vi "HandleObservationSync.vi"(8 "error in (no error)":errorcluster, 11 "S4GUI in":refnum<class "S4GUI.lvclass">) -> (0 "error out":errorcluster, 3 "S4GUI out":refnum<class "S4GUI.lvclass">)   [LabVIEW 2018, in "S4GUI.lvclass"] (continued)
          n1823 = call-dynamic "Read enabled.vi"("error in (no error)"=w5045, "Server in"=w5047) -> ("error out"=w5044:errorcluster, "enabled"=w5043:bool, "Server out"=w5046:refnum<class "Acquisition.lvclass">)  [unwired: 7 in]
          n1824 = case shown="True" w5043 {
            tunnel: [w5101 w5109] -> w5068
            tunnel: [w5102 w5108] -> w5066
            tunnel: w5046 -> [w5102 w5106]
            tunnel: w5044 -> [w5101 w5105]
            frame False {
            }
            frame True {
              n1825 = call-dynamic "Read Channel.vi"("error in (no error)"=w5105, "Acquisition in"=w5106) -> ("error out"=w5113:errorcluster, "Channel.lvclass"=w5114:refnum<class "Channel.lvclass">, "Acquisition out"=w5107:refnum<class "Acquisition.lvclass">)  [unwired: 7 in]
              n1826 = call-dynamic "Read State Machine.vi"("error in (no error)"=w5113, "Device in"=w5114) -> ("error out"=w5112:errorcluster, "State Machine.lvclass"=w5110:refnum<class "State Machine.lvclass">, "Device out"=w5116:refnum<class "Channel.lvclass">)  [unwired: 7 in]
              n1827 = call "Next State.vi"("error in (no error)"=w5112, "New_State"=58, "State Machine in"=w5110) -> ("error out"=w5104:errorcluster, "State Machine out"=w5103:refnum<class "State Machine.lvclass">)  [unwired: 7 in]
              n1828 = call-dynamic "Write State Machine.vi"("error in (no error)"=w5104, "State Machine.lvclass"=w5103, "Device in"=w5116) -> ("error out"=w5117:errorcluster, "Device out"=w5115:refnum<class "Channel.lvclass">)  [unwired: 7 in]
              n1829 = call-dynamic "Write Channel.vi"("error in (no error)"=w5117, "Channel.lvclass"=w5115, "Acquisition in"=w5107) -> ("error out"=w5109:errorcluster, "Acquisition out"=w5108:refnum<class "Acquisition.lvclass">)  [unwired: 7 in]
            }
          }
          n1830 = call-dynamic "Write AcquisitionC.vi"("error in (no error)"=w5068, "Acquisition.lvclass"=w5066, "S4ACS_GUI in"=w5067) -> ("error out"=w5062:errorcluster, "S4ACS_GUI out"=w5061:refnum<class "S4GUI.lvclass">)  [unwired: 7 in]
          n1831 = call-dynamic "Read AcquisitionD.vi"("error in (no error)"=w5062, "S4ACS_GUI in"=w5061) -> ("error out"=w5040:errorcluster, "Acquisition.lvclass"=w5042:refnum<class "Acquisition.lvclass">, "S4ACS_GUI out"=w5060:refnum<class "S4GUI.lvclass">)  [unwired: 7 in]
          n1832 = call-dynamic "Read enabled.vi"("error in (no error)"=w5040, "Server in"=w5042) -> ("error out"=w5039:errorcluster, "enabled"=w5038:bool, "Server out"=w5041:refnum<class "Acquisition.lvclass">)  [unwired: 7 in]
          n1833 = case shown="True" w5038 {
            tunnel: w5039 -> [w5084 w5100]
            tunnel: [w5084 w5099] -> w5063
            tunnel: w5041 -> [w5085 w5090]
            tunnel: [w5085 w5088] -> w5059
            frame False {
            }
            frame True {
              n1834 = call-dynamic "Read Channel.vi"("error in (no error)"=w5100, "Acquisition in"=w5090) -> ("error out"=w5095:errorcluster, "Channel.lvclass"=w5094:refnum<class "Channel.lvclass">, "Acquisition out"=w5089:refnum<class "Acquisition.lvclass">)  [unwired: 7 in]
              n1835 = call-dynamic "Read State Machine.vi"("error in (no error)"=w5095, "Device in"=w5094) -> ("error out"=w5096:errorcluster, "State Machine.lvclass"=w5098:refnum<class "State Machine.lvclass">, "Device out"=w5092:refnum<class "Channel.lvclass">)  [unwired: 7 in]
              n1836 = call "Next State.vi"("error in (no error)"=w5096, "New_State"=58, "State Machine in"=w5098) -> ("error out"=w5086:errorcluster, "State Machine out"=w5087:refnum<class "State Machine.lvclass">)  [unwired: 7 in]
              n1837 = call-dynamic "Write State Machine.vi"("error in (no error)"=w5086, "State Machine.lvclass"=w5087, "Device in"=w5092) -> ("error out"=w5091:errorcluster, "Device out"=w5093:refnum<class "Channel.lvclass">)  [unwired: 7 in]
              n1838 = call-dynamic "Write Channel.vi"("error in (no error)"=w5091, "Channel.lvclass"=w5093, "Acquisition in"=w5089) -> ("error out"=w5099:errorcluster, "Acquisition out"=w5088:refnum<class "Acquisition.lvclass">)  [unwired: 7 in]
            }
          }
          n1839 = call-dynamic "Write AcquisitionD.vi"("error in (no error)"=w5063, "Acquisition.lvclass"=w5059, "S4ACS_GUI in"=w5060) -> ("error out"=w5037:errorcluster, "S4ACS_GUI out"=w5058:refnum<class "S4GUI.lvclass">)  [unwired: 7 in]
          n1840 = flat-sequence {
            tunnel: w5037 -> [w5082]
            tunnel: [w5082] -> w5036
            frame #0 {
              n1841 = Tick Count (ms)() -> (millisecond timer value=→"time9":u32)
            }
          }
          n1842 = Increment(x=w5076) -> (x+1=w5075:u32)
          n1843 = Bundle By Name(cluster=w5058, "Obs_state"=w5075) -> (w5074:refnum<class "S4GUI.lvclass">)
        }
        frame 363 {
          # "T: mode EXPOSE\nF: mode FIRE\nNa seq de foco, só \ndeve usar mode EXPOSE."
          # "Espera todos os canais chegarem ao estado de repouso.\n(estado 0  de Channel:Run.vi)."
          n1844 = call-dynamic "Read AcquisitionA.vi"("error in (no error)"=w5202, "S4ACS_GUI in"=w5203) -> ("error out"=w5181:errorcluster, "Acquisition.lvclass"=w5182:refnum<class "Acquisition.lvclass">, "S4ACS_GUI out"=w5205:refnum<class "S4GUI.lvclass">)  [unwired: 7 in]
          n1845 = call-dynamic "Read enabled.vi"("error in (no error)"=w5181, "Server in"=w5182) -> ("error out"=w5183:errorcluster, "enabled"=w5185:bool, "Server out"=w5184:refnum<class "Acquisition.lvclass">)  [unwired: 7 in]
          n1846 = case shown="True" w5185 {
            tunnel: [w5279 w5297] -> w5206
            tunnel: [w5278 w5296] -> w5204
            tunnel: w5184 -> [w5279 w5289]
            tunnel: w5183 -> [w5278 w5288]
            tunnel: [TRUE w5281] -> w5162
            tunnel: [FALSE w5282] -> w5158
            frame False {
            }
            frame True {
              n1847 = call-dynamic "Read Channel.vi"("error in (no error)"=w5288, "Acquisition in"=w5289) -> ("error out"=w5285:errorcluster, "Channel.lvclass"=w5286:refnum<class "Channel.lvclass">, "Acquisition out"=w5298:refnum<class "Acquisition.lvclass">)  [unwired: 7 in]
              n1848 = call-dynamic "Read wait_expose.vi"("error in (no error)"=w5285, "Channel in"=w5286) -> ("error out"=w5283:errorcluster, "wait_expose"=w5282:bool, "Channel out"=w5284:refnum<class "Channel.lvclass">)  [unwired: 7 in]
              n1849 = call-dynamic "Read State Machine.vi"("error in (no error)"=w5283, "Device in"=w5284) -> ("error out"=w5290:errorcluster, "State Machine.lvclass"=w5292:refnum<class "State Machine.lvclass">, "Device out"=w5294:refnum<class "Channel.lvclass">)  [unwired: 7 in]
              n1850 = call-dynamic "Read State.vi"("error in (no error)"=w5290, "State Machine in"=w5292) -> ("error out"=w5287:errorcluster, "State"=w5280:i32, "State Machine out"=w5291:refnum<class "State Machine.lvclass">)  [unwired: 7 in]
              n1851 = Equal To 0?(x=w5280) -> (x = 0?=w5281:bool)
              n1852 = call-dynamic "Write State Machine.vi"("error in (no error)"=w5287, "State Machine.lvclass"=w5291, "Device in"=w5294) -> ("error out"=w5293:errorcluster, "Device out"=w5295:refnum<class "Channel.lvclass">)  [unwired: 7 in]
              n1853 = call-dynamic "Write Channel.vi"("error in (no error)"=w5293, "Channel.lvclass"=w5295, "Acquisition in"=w5298) -> ("error out"=w5296:errorcluster, "Acquisition out"=w5297:refnum<class "Acquisition.lvclass">)  [unwired: 7 in]
            }
          }
          n1854 = call-dynamic "Write AcquisitionA.vi"("error in (no error)"=w5204, "Acquisition.lvclass"=w5206, "S4ACS_GUI in"=w5205) -> ("error out"=w5198:errorcluster, "S4ACS_GUI out"=w5199:refnum<class "S4GUI.lvclass">)  [unwired: 7 in]
          n1855 = call "Read AcquisitionB.vi"("error in (no error)"=w5198, "S4ACS_GUI in"=w5199) -> ("error out"=w5178:errorcluster, "Acquisition.lvclass"=w5180:refnum<class "Acquisition.lvclass">, "S4ACS_GUI out"=w5196:refnum<class "S4GUI.lvclass">)  [unwired: 7 in]
          n1856 = call-dynamic "Read enabled.vi"("error in (no error)"=w5178, "Server in"=w5180) -> ("error out"=w5177:errorcluster, "enabled"=w5176:bool, "Server out"=w5179:refnum<class "Acquisition.lvclass">)  [unwired: 7 in]
          n1857 = case shown="True" w5176 {
            tunnel: w5179 -> [w5256 w5275]
            tunnel: w5177 -> [w5255 w5274]
            tunnel: [w5256 w5272] -> w5197
            tunnel: [w5255 w5271] -> w5195
            tunnel: [TRUE w5263] -> w5161
            tunnel: [FALSE ("expose") w5257] -> w5157
            frame False {
            }
            frame True {
              n1858 = call-dynamic "Read Channel.vi"("error in (no error)"=w5274, "Acquisition in"=w5275) -> ("error out"=w5259:errorcluster, "Channel.lvclass"=w5261:refnum<class "Channel.lvclass">, "Acquisition out"=w5273:refnum<class "Acquisition.lvclass">)  [unwired: 7 in]
              n1859 = call-dynamic "Read wait_expose.vi"("error in (no error)"=w5259, "Channel in"=w5261) -> ("error out"=w5258:errorcluster, "wait_expose"=w5257:bool, "Channel out"=w5260:refnum<class "Channel.lvclass">)  [unwired: 7 in]
              n1860 = call-dynamic "Read State Machine.vi"("error in (no error)"=w5258, "Device in"=w5260) -> ("error out"=w5265:errorcluster, "State Machine.lvclass"=w5267:refnum<class "State Machine.lvclass">, "Device out"=w5269:refnum<class "Channel.lvclass">)  [unwired: 7 in]
              n1861 = call-dynamic "Read State.vi"("error in (no error)"=w5265, "State Machine in"=w5267) -> ("error out"=w5264:errorcluster, "State"=w5262:i32, "State Machine out"=w5266:refnum<class "State Machine.lvclass">)  [unwired: 7 in]
              n1862 = Equal To 0?(x=w5262) -> (x = 0?=w5263:bool)
              n1863 = call-dynamic "Write State Machine.vi"("error in (no error)"=w5264, "State Machine.lvclass"=w5266, "Device in"=w5269) -> ("error out"=w5268:errorcluster, "Device out"=w5270:refnum<class "Channel.lvclass">)  [unwired: 7 in]
              n1864 = call-dynamic "Write Channel.vi"("error in (no error)"=w5268, "Channel.lvclass"=w5270, "Acquisition in"=w5273) -> ("error out"=w5271:errorcluster, "Acquisition out"=w5272:refnum<class "Acquisition.lvclass">)  [unwired: 7 in]
            }
          }
          n1865 = call "Write AcquisitionB.vi"("error in (no error)"=w5195, "Acquisition.lvclass"=w5197, "S4ACS_GUI in"=w5196) -> ("error out"=w5191:errorcluster, "S4ACS_GUI out"=w5190:refnum<class "S4GUI.lvclass">)  [unwired: 7 in]
          n1866 = call-dynamic "Read AcquisitionC.vi"("error in (no error)"=w5191, "S4ACS_GUI in"=w5190) -> ("error out"=w5173:errorcluster, "Acquisition.lvclass"=w5175:refnum<class "Acquisition.lvclass">, "S4ACS_GUI out"=w5193:refnum<class "S4GUI.lvclass">)  [unwired: 7 in]
          n1867 = call-dynamic "Read enabled.vi"("error in (no error)"=w5173, "Server in"=w5175) -> ("error out"=w5172:errorcluster, "enabled"=w5171:bool, "Server out"=w5174:refnum<class "Acquisition.lvclass">)  [unwired: 7 in]
          n1868 = case shown="True" w5171 {
            tunnel: [w5232 w5247] -> w5194
            tunnel: [w5233 w5246] -> w5192
            tunnel: w5174 -> [w5233 w5242]
            tunnel: w5172 -> [w5232 w5241]
            tunnel: [TRUE w5239] -> w5160
            tunnel: [FALSE ("expose") w5234] -> w5156
            frame False {
            }
            frame True {
              n1869 = call-dynamic "Read Channel.vi"("error in (no error)"=w5241, "Acquisition in"=w5242) -> ("error out"=w5236:errorcluster, "Channel.lvclass"=w5238:refnum<class "Channel.lvclass">, "Acquisition out"=w5245:refnum<class "Acquisition.lvclass">)  [unwired: 7 in]
              n1870 = call-dynamic "Read wait_expose.vi"("error in (no error)"=w5236, "Channel in"=w5238) -> ("error out"=w5235:errorcluster, "wait_expose"=w5234:bool, "Channel out"=w5237:refnum<class "Channel.lvclass">)  [unwired: 7 in]
              n1871 = call-dynamic "Read State Machine.vi"("error in (no error)"=w5235, "Device in"=w5237) -> ("error out"=w5243:errorcluster, "State Machine.lvclass"=w5251:refnum<class "State Machine.lvclass">, "Device out"=w5249:refnum<class "Channel.lvclass">)  [unwired: 7 in]
              n1872 = call-dynamic "Read State.vi"("error in (no error)"=w5243, "State Machine in"=w5251) -> ("error out"=w5244:errorcluster, "State"=w5240:i32, "State Machine out"=w5252:refnum<class "State Machine.lvclass">)  [unwired: 7 in]
              n1873 = Equal To 0?(x=w5240) -> (x = 0?=w5239:bool)
              n1874 = call-dynamic "Write State Machine.vi"("error in (no error)"=w5244, "State Machine.lvclass"=w5252, "Device in"=w5249) -> ("error out"=w5250:errorcluster, "Device out"=w5248:refnum<class "Channel.lvclass">)  [unwired: 7 in]
              n1875 = call-dynamic "Write Channel.vi"("error in (no error)"=w5250, "Channel.lvclass"=w5248, "Acquisition in"=w5245) -> ("error out"=w5247:errorcluster, "Acquisition out"=w5246:refnum<class "Acquisition.lvclass">)  [unwired: 7 in]
            }
          }
          n1876 = call-dynamic "Write AcquisitionC.vi"("error in (no error)"=w5194, "Acquisition.lvclass"=w5192, "S4ACS_GUI in"=w5193) -> ("error out"=w5170:errorcluster, "S4ACS_GUI out"=w5186:refnum<class "S4GUI.lvclass">)  [unwired: 7 in]
          n1877 = call-dynamic "Read AcquisitionD.vi"("error in (no error)"=w5170, "S4ACS_GUI in"=w5186) -> ("error out"=w5166:errorcluster, "Acquisition.lvclass"=w5169:refnum<class "Acquisition.lvclass">, "S4ACS_GUI out"=w5188:refnum<class "S4GUI.lvclass">)  [unwired: 7 in]
          n1878 = call-dynamic "Read enabled.vi"("error in (no error)"=w5166, "Server in"=w5169) -> ("error out"=w5167:errorcluster, "enabled"=w5165:bool, "Server out"=w5168:refnum<class "Acquisition.lvclass">)  [unwired: 7 in]
          n1879 = case shown="True" w5165 {
            tunnel: [w5210 w5228] -> w5189
            tunnel: [w5209 w5227] -> w5187
            tunnel: [TRUE w5217] -> w5159
            tunnel: w5168 -> [w5210 w5219]
            tunnel: w5167 -> [w5209 w5218]
            tunnel: [FALSE ("expose") w5211] -> w5155
            frame False {
            }
            frame True {
              n1880 = call-dynamic "Read Channel.vi"("error in (no error)"=w5218, "Acquisition in"=w5219) -> ("error out"=w5213:errorcluster, "Channel.lvclass"=w5215:refnum<class "Channel.lvclass">, "Acquisition out"=w5229:refnum<class "Acquisition.lvclass">)  [unwired: 7 in]
              n1881 = call-dynamic "Read wait_expose.vi"("error in (no error)"=w5213, "Channel in"=w5215) -> ("error out"=w5212:errorcluster, "wait_expose"=w5211:bool, "Channel out"=w5214:refnum<class "Channel.lvclass">)  [unwired: 7 in]
              n1882 = call-dynamic "Read State Machine.vi"("error in (no error)"=w5212, "Device in"=w5214) -> ("error out"=w5221:errorcluster, "State Machine.lvclass"=w5223:refnum<class "State Machine.lvclass">, "Device out"=w5225:refnum<class "Channel.lvclass">)  [unwired: 7 in]
              n1883 = call-dynamic "Read State.vi"("error in (no error)"=w5221, "State Machine in"=w5223) -> ("error out"=w5220:errorcluster, "State"=w5216:i32, "State Machine out"=w5222:refnum<class "State Machine.lvclass">)  [unwired: 7 in]
              n1884 = Equal To 0?(x=w5216) -> (x = 0?=w5217:bool)
              n1885 = call-dynamic "Write State Machine.vi"("error in (no error)"=w5220, "State Machine.lvclass"=w5222, "Device in"=w5225) -> ("error out"=w5224:errorcluster, "Device out"=w5226:refnum<class "Channel.lvclass">)  [unwired: 7 in]
              n1886 = call-dynamic "Write Channel.vi"("error in (no error)"=w5224, "Channel.lvclass"=w5226, "Acquisition in"=w5229) -> ("error out"=w5227:errorcluster, "Acquisition out"=w5228:refnum<class "Acquisition.lvclass">)  [unwired: 7 in]
            }
          }
          n1887 = call-dynamic "Write AcquisitionD.vi"("error in (no error)"=w5187, "Acquisition.lvclass"=w5189, "S4ACS_GUI in"=w5188) -> ("error out"=w5153:errorcluster, "S4ACS_GUI out"=w5154:refnum<class "S4GUI.lvclass">)  [unwired: 7 in]
          n1888 = Compound Arithmetic op=OR(w5158, w5157, w5156, w5155) -> ()  [unwired: 1 out]
          n1889 = Compound Arithmetic op=AND(w5162, w5161, w5160, w5159) -> (w5163:bool)
          n1890 = Increment(x=w5164) -> (x+1=w5152:u32)
          n1891 = Select(t=w5152, s=w5163, f=w5164) -> (s? t:f=w5200:u32)
          n1892 = Bundle By Name(cluster=w5154, "Obs_state"=w5200) -> (w5201:refnum<class "S4GUI.lvclass">)
        }
        frame 364 {
          n1893 = flat-sequence {
            tunnel: [w5312] -> w5300
            tunnel: w5301 -> [w5312]
            tunnel: [w5308] -> w5299
            frame #0 {
              # "Espera 2s desde que enviou o comando\nWRITE_HEADER_DATA para os ACS"
              n1894 = local read "time9"() -> (w5307:u32)
              n1895 = Tick Count (ms)() -> (millisecond timer value=w5311:u32)
              "time 10" <- w5311
              n1896 = Subtract(x=w5311, y=w5307) -> (x-y=w5310:u32)
              "delay 89" <- w5310
              n1897 = Greater?(x=w5310, y=u32 2000) -> (0:w5308:bool)
            }
          }
          n1898 = Increment(x=w5304) -> (x+1=w5303:u32)
          n1899 = Select(t=w5303, s=w5299, f=w5304) -> (s? t:f=w5305:u32)
          n1900 = Bundle By Name(cluster=w5302, "Obs_state"=w5305) -> (w5306:refnum<class "S4GUI.lvclass">)
        }
        frame 365 {
          n1901 = call-dynamic "Read AcquisitionA.vi"("error in (no error)"=w5353, "S4ACS_GUI in"=w5354) -> ("error out"=w5329:errorcluster, "Acquisition.lvclass"=w5332:refnum<class "Acquisition.lvclass">, "S4ACS_GUI out"=w5356:refnum<class "S4GUI.lvclass">)  [unwired: 7 in]
          n1902 = call-dynamic "Read enabled.vi"("error in (no error)"=w5329, "Server in"=w5332) -> ("error out"=w5328:errorcluster, "enabled"=w5330:bool, "Server out"=w5331:refnum<class "Acquisition.lvclass">)  [unwired: 7 in]
          n1903 = case shown="True" w5330 {
            tunnel: w5331 -> [w5410 w5425]
            tunnel: w5328 -> [w5409 w5424]
            tunnel: [w5410 w5422] -> w5357
            tunnel: [w5409 w5421] -> w5355
            frame False {
            }
            frame True {
              n1904 = call-dynamic "Read Channel.vi"("error in (no error)"=w5424, "Acquisition in"=w5425) -> ("error out"=w5417:errorcluster, "Channel.lvclass"=w5416:refnum<class "Channel.lvclass">, "Acquisition out"=w5423:refnum<class "Acquisition.lvclass">)  [unwired: 7 in]
              n1905 = call-dynamic "Read State Machine.vi"("error in (no error)"=w5417, "Device in"=w5416) -> ("error out"=w5418:errorcluster, "State Machine.lvclass"=w5420:refnum<class "State Machine.lvclass">, "Device out"=w5414:refnum<class "Channel.lvclass">)  [unwired: 7 in]
              n1906 = call "Next State.vi"("error in (no error)"=w5418, "New_State"=50, "State Machine in"=w5420) -> ("error out"=w5411:errorcluster, "State Machine out"=w5412:refnum<class "State Machine.lvclass">)  [unwired: 7 in]
              n1907 = call-dynamic "Write State Machine.vi"("error in (no error)"=w5411, "State Machine.lvclass"=w5412, "Device in"=w5414) -> ("error out"=w5413:errorcluster, "Device out"=w5415:refnum<class "Channel.lvclass">)  [unwired: 7 in]
              n1908 = call-dynamic "Write Channel.vi"("error in (no error)"=w5413, "Channel.lvclass"=w5415, "Acquisition in"=w5423) -> ("error out"=w5421:errorcluster, "Acquisition out"=w5422:refnum<class "Acquisition.lvclass">)  [unwired: 7 in]
            }
          }
          n1909 = call-dynamic "Write AcquisitionA.vi"("error in (no error)"=w5355, "Acquisition.lvclass"=w5357, "S4ACS_GUI in"=w5356) -> ("error out"=w5348:errorcluster, "S4ACS_GUI out"=w5349:refnum<class "S4GUI.lvclass">)  [unwired: 7 in]
          n1910 = call "Read AcquisitionB.vi"("error in (no error)"=w5348, "S4ACS_GUI in"=w5349) -> ("error out"=w5325:errorcluster, "Acquisition.lvclass"=w5327:refnum<class "Acquisition.lvclass">, "S4ACS_GUI out"=w5346:refnum<class "S4GUI.lvclass">)  [unwired: 7 in]
          n1911 = call-dynamic "Read enabled.vi"("error in (no error)"=w5325, "Server in"=w5327) -> ("error out"=w5324:errorcluster, "enabled"=w5323:bool, "Server out"=w5326:refnum<class "Acquisition.lvclass">)  [unwired: 7 in]
          n1912 = case shown="True" w5323 {
            tunnel: w5326 -> [w5393 w5408]
            tunnel: w5324 -> [w5392 w5407]
            tunnel: [w5393 w5405] -> w5347
            tunnel: [w5392 w5404] -> w5345
            frame False {
            }
            frame True {
              n1913 = call-dynamic "Read Channel.vi"("error in (no error)"=w5407, "Acquisition in"=w5408) -> ("error out"=w5400:errorcluster, "Channel.lvclass"=w5399:refnum<class "Channel.lvclass">, "Acquisition out"=w5406:refnum<class "Acquisition.lvclass">)  [unwired: 7 in]
              n1914 = call-dynamic "Read State Machine.vi"("error in (no error)"=w5400, "Device in"=w5399) -> ("error out"=w5401:errorcluster, "State Machine.lvclass"=w5403:refnum<class "State Machine.lvclass">, "Device out"=w5397:refnum<class "Channel.lvclass">)  [unwired: 7 in]
              n1915 = call "Next State.vi"("error in (no error)"=w5401, "New_State"=50, "State Machine in"=w5403) -> ("error out"=w5394:errorcluster, "State Machine out"=w5395:refnum<class "State Machine.lvclass">)  [unwired: 7 in]
              n1916 = call-dynamic "Write State Machine.vi"("error in (no error)"=w5394, "State Machine.lvclass"=w5395, "Device in"=w5397) -> ("error out"=w5396:errorcluster, "Device out"=w5398:refnum<class "Channel.lvclass">)  [unwired: 7 in]
              n1917 = call-dynamic "Write Channel.vi"("error in (no error)"=w5396, "Channel.lvclass"=w5398, "Acquisition in"=w5406) -> ("error out"=w5404:errorcluster, "Acquisition out"=w5405:refnum<class "Acquisition.lvclass">)  [unwired: 7 in]
            }
          }
          n1918 = call "Write AcquisitionB.vi"("error in (no error)"=w5345, "Acquisition.lvclass"=w5347, "S4ACS_GUI in"=w5346) -> ("error out"=w5341:errorcluster, "S4ACS_GUI out"=w5340:refnum<class "S4GUI.lvclass">)  [unwired: 7 in]
          n1919 = call-dynamic "Read AcquisitionC.vi"("error in (no error)"=w5341, "S4ACS_GUI in"=w5340) -> ("error out"=w5320:errorcluster, "Acquisition.lvclass"=w5322:refnum<class "Acquisition.lvclass">, "S4ACS_GUI out"=w5343:refnum<class "S4GUI.lvclass">)  [unwired: 7 in]
          n1920 = call-dynamic "Read enabled.vi"("error in (no error)"=w5320, "Server in"=w5322) -> ("error out"=w5319:errorcluster, "enabled"=w5318:bool, "Server out"=w5321:refnum<class "Acquisition.lvclass">)  [unwired: 7 in]
          n1921 = case shown="True" w5318 {
            tunnel: [w5375 w5383] -> w5344
            tunnel: [w5376 w5382] -> w5342
            tunnel: w5321 -> [w5376 w5380]
            tunnel: w5319 -> [w5375 w5379]
            frame False {
            }
            frame True {
              n1922 = call-dynamic "Read Channel.vi"("error in (no error)"=w5379, "Acquisition in"=w5380) -> ("error out"=w5387:errorcluster, "Channel.lvclass"=w5388:refnum<class "Channel.lvclass">, "Acquisition out"=w5381:refnum<class "Acquisition.lvclass">)  [unwired: 7 in]
              n1923 = call-dynamic "Read State Machine.vi"("error in (no error)"=w5387, "Device in"=w5388) -> ("error out"=w5386:errorcluster, "State Machine.lvclass"=w5384:refnum<class "State Machine.lvclass">, "Device out"=w5390:refnum<class "Channel.lvclass">)  [unwired: 7 in]
              n1924 = call "Next State.vi"("error in (no error)"=w5386, "New_State"=50, "State Machine in"=w5384) -> ("error out"=w5378:errorcluster, "State Machine out"=w5377:refnum<class "State Machine.lvclass">)  [unwired: 7 in]
              n1925 = call-dynamic "Write State Machine.vi"("error in (no error)"=w5378, "State Machine.lvclass"=w5377, "Device in"=w5390) -> ("error out"=w5391:errorcluster, "Device out"=w5389:refnum<class "Channel.lvclass">)  [unwired: 7 in]
              n1926 = call-dynamic "Write Channel.vi"("error in (no error)"=w5391, "Channel.lvclass"=w5389, "Acquisition in"=w5381) -> ("error out"=w5383:errorcluster, "Acquisition out"=w5382:refnum<class "Acquisition.lvclass">)  [unwired: 7 in]
            }
          }
          n1927 = call-dynamic "Write AcquisitionC.vi"("error in (no error)"=w5344, "Acquisition.lvclass"=w5342, "S4ACS_GUI in"=w5343) -> ("error out"=w5338:errorcluster, "S4ACS_GUI out"=w5337:refnum<class "S4GUI.lvclass">)  [unwired: 7 in]
          n1928 = call-dynamic "Read AcquisitionD.vi"("error in (no error)"=w5338, "S4ACS_GUI in"=w5337) -> ("error out"=w5315:errorcluster, "Acquisition.lvclass"=w5317:refnum<class "Acquisition.lvclass">, "S4ACS_GUI out"=w5336:refnum<class "S4GUI.lvclass">)  [unwired: 7 in]
          n1929 = call-dynamic "Read enabled.vi"("error in (no error)"=w5315, "Server in"=w5317) -> ("error out"=w5314:errorcluster, "enabled"=w5313:bool, "Server out"=w5316:refnum<class "Acquisition.lvclass">)  [unwired: 7 in]
          n1930 = case shown="True" w5313 {
            tunnel: w5314 -> [w5358 w5374]
            tunnel: [w5358 w5373] -> w5339
            tunnel: w5316 -> [w5359 w5364]
            tunnel: [w5359 w5362] -> w5335
            frame False {
            }
            frame True {
              n1931 = call-dynamic "Read Channel.vi"("error in (no error)"=w5374, "Acquisition in"=w5364) -> ("error out"=w5369:errorcluster, "Channel.lvclass"=w5368:refnum<class "Channel.lvclass">, "Acquisition out"=w5363:refnum<class "Acquisition.lvclass">)  [unwired: 7 in]
              n1932 = call-dynamic "Read State Machine.vi"("error in (no error)"=w5369, "Device in"=w5368) -> ("error out"=w5370:errorcluster, "State Machine.lvclass"=w5372:refnum<class "State Machine.lvclass">, "Device out"=w5366:refnum<class "Channel.lvclass">)  [unwired: 7 in]
              n1933 = call "Next State.vi"("error in (no error)"=w5370, "New_State"=50, "State Machine in"=w5372) -> ("error out"=w5360:errorcluster, "State Machine out"=w5361:refnum<class "State Machine.lvclass">)  [unwired: 7 in]
              n1934 = call-dynamic "Write State Machine.vi"("error in (no error)"=w5360, "State Machine.lvclass"=w5361, "Device in"=w5366) -> ("error out"=w5365:errorcluster, "Device out"=w5367:refnum<class "Channel.lvclass">)  [unwired: 7 in]
              n1935 = call-dynamic "Write Channel.vi"("error in (no error)"=w5365, "Channel.lvclass"=w5367, "Acquisition in"=w5363) -> ("error out"=w5373:errorcluster, "Acquisition out"=w5362:refnum<class "Acquisition.lvclass">)  [unwired: 7 in]
            }
          }
          n1936 = call-dynamic "Write AcquisitionD.vi"("error in (no error)"=w5339, "Acquisition.lvclass"=w5335, "S4ACS_GUI in"=w5336) -> ("error out"=w5334:errorcluster, "S4ACS_GUI out"=w5333:refnum<class "S4GUI.lvclass">)  [unwired: 7 in]
          n1937 = Increment(x=w5352) -> (x+1=w5351:u32)
          n1938 = Bundle By Name(cluster=w5333, "Obs_state"=w5351) -> (w5350:refnum<class "S4GUI.lvclass">)
        }
        frame 366 {
          # "Espera todos os canais com CyclesDone=0"
          # "Espera todos os canais chegarem ao estado ACTIVE\n(estados 54 e 55 de Channel:Run.vi)."
          n1939 = call-dynamic "Read AcquisitionA.vi"("error in (no error)"=w5477, "S4ACS_GUI in"=w5478) -> ("error out"=w5456:errorcluster, "Acquisition.lvclass"=w5457:refnum<class "Acquisition.lvclass">, "S4ACS_GUI out"=w5480:refnum<class "S4GUI.lvclass">)  [unwired: 7 in]
          n1940 = call-dynamic "Read enabled.vi"("error in (no error)"=w5456, "Server in"=w5457) -> ("error out"=w5458:errorcluster, "enabled"=w5460:bool, "Server out"=w5459:refnum<class "Acquisition.lvclass">)  [unwired: 7 in]
          n1941 = case shown="True" w5460 {
            tunnel: [w5557 w5576] -> w5481
            tunnel: [w5556 w5575] -> w5479
            tunnel: w5459 -> [w5557 w5568]
            tunnel: w5458 -> [w5556 w5567]
            tunnel: [TRUE w5566] -> w5438
            tunnel: [u32 0 ("CyclesDone") w5558] -> w5430
            frame False {
            }
            frame True {
              n1942 = call-dynamic "Read Channel.vi"("error in (no error)"=w5567, "Acquisition in"=w5568) -> ("error out"=w5561:errorcluster, "Channel.lvclass"=w5562:refnum<class "Channel.lvclass">, "Acquisition out"=w5577:refnum<class "Acquisition.lvclass">)  [unwired: 7 in]
              n1943 = call-dynamic "Read CyclesDone.vi"("error in (no error)"=w5561, "Channel in"=w5562) -> ("error out"=w5559:errorcluster, "CyclesDone"=w5558:u32, "Channel out"=w5560:refnum<class "Channel.lvclass">)  [unwired: 7 in]
              n1944 = call-dynamic "Read State Machine.vi"("error in (no error)"=w5559, "Device in"=w5560) -> ("error out"=w5569:errorcluster, "State Machine.lvclass"=w5571:refnum<class "State Machine.lvclass">, "Device out"=w5573:refnum<class "Channel.lvclass">)  [unwired: 7 in]
              n1945 = call-dynamic "Read State.vi"("error in (no error)"=w5569, "State Machine in"=w5571) -> ("error out"=w5563:errorcluster, "State"=w5565:i32, "State Machine out"=w5570:refnum<class "State Machine.lvclass">)  [unwired: 7 in]
              n1946 = Greater?(x=w5565, y=53) -> (0:w5566:bool)
              n1947 = call-dynamic "Write State Machine.vi"("error in (no error)"=w5563, "State Machine.lvclass"=w5570, "Device in"=w5573) -> ("error out"=w5572:errorcluster, "Device out"=w5574:refnum<class "Channel.lvclass">)  [unwired: 7 in]
              n1948 = call-dynamic "Write Channel.vi"("error in (no error)"=w5572, "Channel.lvclass"=w5574, "Acquisition in"=w5577) -> ("error out"=w5575:errorcluster, "Acquisition out"=w5576:refnum<class "Acquisition.lvclass">)  [unwired: 7 in]
            }
          }
          n1949 = call-dynamic "Write AcquisitionA.vi"("error in (no error)"=w5479, "Acquisition.lvclass"=w5481, "S4ACS_GUI in"=w5480) -> ("error out"=w5473:errorcluster, "S4ACS_GUI out"=w5474:refnum<class "S4GUI.lvclass">)  [unwired: 7 in]
          n1950 = call "Read AcquisitionB.vi"("error in (no error)"=w5473, "S4ACS_GUI in"=w5474) -> ("error out"=w5453:errorcluster, "Acquisition.lvclass"=w5455:refnum<class "Acquisition.lvclass">, "S4ACS_GUI out"=w5471:refnum<class "S4GUI.lvclass">)  [unwired: 7 in]
          n1951 = call-dynamic "Read enabled.vi"("error in (no error)"=w5453, "Server in"=w5455) -> ("error out"=w5452:errorcluster, "enabled"=w5451:bool, "Server out"=w5454:refnum<class "Acquisition.lvclass">)  [unwired: 7 in]
          n1952 = case shown="True" w5451 {
            tunnel: w5454 -> [w5533 w5553]
            tunnel: w5452 -> [w5532 w5552]
            tunnel: [w5533 w5550] -> w5472
            tunnel: [w5532 w5549] -> w5470
            tunnel: [TRUE w5540] -> w5437
            tunnel: [u32 0 ("CyclesDone") w5534] -> w5431
            frame False {
            }
            frame True {
              n1953 = call-dynamic "Read Channel.vi"("error in (no error)"=w5552, "Acquisition in"=w5553) -> ("error out"=w5536:errorcluster, "Channel.lvclass"=w5538:refnum<class "Channel.lvclass">, "Acquisition out"=w5551:refnum<class "Acquisition.lvclass">)  [unwired: 7 in]
              n1954 = call-dynamic "Read CyclesDone.vi"("error in (no error)"=w5536, "Channel in"=w5538) -> ("error out"=w5535:errorcluster, "CyclesDone"=w5534:u32, "Channel out"=w5537:refnum<class "Channel.lvclass">)  [unwired: 7 in]
              n1955 = call-dynamic "Read State Machine.vi"("error in (no error)"=w5535, "Device in"=w5537) -> ("error out"=w5543:errorcluster, "State Machine.lvclass"=w5545:refnum<class "State Machine.lvclass">, "Device out"=w5547:refnum<class "Channel.lvclass">)  [unwired: 7 in]
              n1956 = call-dynamic "Read State.vi"("error in (no error)"=w5543, "State Machine in"=w5545) -> ("error out"=w5542:errorcluster, "State"=w5539:i32, "State Machine out"=w5544:refnum<class "State Machine.lvclass">)  [unwired: 7 in]
              n1957 = Greater?(x=w5539, y=53) -> (0:w5540:bool)
              n1958 = call-dynamic "Write State Machine.vi"("error in (no error)"=w5542, "State Machine.lvclass"=w5544, "Device in"=w5547) -> ("error out"=w5546:errorcluster, "Device out"=w5548:refnum<class "Channel.lvclass">)  [unwired: 7 in]
              n1959 = call-dynamic "Write Channel.vi"("error in (no error)"=w5546, "Channel.lvclass"=w5548, "Acquisition in"=w5551) -> ("error out"=w5549:errorcluster, "Acquisition out"=w5550:refnum<class "Acquisition.lvclass">)  [unwired: 7 in]
            }
          }
          n1960 = call "Write AcquisitionB.vi"("error in (no error)"=w5470, "Acquisition.lvclass"=w5472, "S4ACS_GUI in"=w5471) -> ("error out"=w5466:errorcluster, "S4ACS_GUI out"=w5465:refnum<class "S4GUI.lvclass">)  [unwired: 7 in]
          n1961 = call-dynamic "Read AcquisitionC.vi"("error in (no error)"=w5466, "S4ACS_GUI in"=w5465) -> ("error out"=w5448:errorcluster, "Acquisition.lvclass"=w5450:refnum<class "Acquisition.lvclass">, "S4ACS_GUI out"=w5468:refnum<class "S4GUI.lvclass">)  [unwired: 7 in]
          n1962 = call-dynamic "Read enabled.vi"("error in (no error)"=w5448, "Server in"=w5450) -> ("error out"=w5447:errorcluster, "enabled"=w5446:bool, "Server out"=w5449:refnum<class "Acquisition.lvclass">)  [unwired: 7 in]
          n1963 = case shown="True" w5446 {
            tunnel: [w5508 w5524] -> w5469
            tunnel: [w5509 w5523] -> w5467
            tunnel: w5449 -> [w5509 w5519]
            tunnel: w5447 -> [w5508 w5518]
            tunnel: [TRUE w5515] -> w5436
            tunnel: [u32 0 ("CyclesDone") w5510] -> w5429
            frame False {
            }
            frame True {
              n1964 = call-dynamic "Read Channel.vi"("error in (no error)"=w5518, "Acquisition in"=w5519) -> ("error out"=w5512:errorcluster, "Channel.lvclass"=w5514:refnum<class "Channel.lvclass">, "Acquisition out"=w5522:refnum<class "Acquisition.lvclass">)  [unwired: 7 in]
              n1965 = call-dynamic "Read CyclesDone.vi"("error in (no error)"=w5512, "Channel in"=w5514) -> ("error out"=w5511:errorcluster, "CyclesDone"=w5510:u32, "Channel out"=w5513:refnum<class "Channel.lvclass">)  [unwired: 7 in]
              n1966 = call-dynamic "Read State Machine.vi"("error in (no error)"=w5511, "Device in"=w5513) -> ("error out"=w5520:errorcluster, "State Machine.lvclass"=w5528:refnum<class "State Machine.lvclass">, "Device out"=w5526:refnum<class "Channel.lvclass">)  [unwired: 7 in]
              n1967 = call-dynamic "Read State.vi"("error in (no error)"=w5520, "State Machine in"=w5528) -> ("error out"=w5521:errorcluster, "State"=w5516:i32, "State Machine out"=w5529:refnum<class "State Machine.lvclass">)  [unwired: 7 in]
              n1968 = Greater?(x=w5516, y=53) -> (0:w5515:bool)
              n1969 = call-dynamic "Write State Machine.vi"("error in (no error)"=w5521, "State Machine.lvclass"=w5529, "Device in"=w5526) -> ("error out"=w5527:errorcluster, "Device out"=w5525:refnum<class "Channel.lvclass">)  [unwired: 7 in]
              n1970 = call-dynamic "Write Channel.vi"("error in (no error)"=w5527, "Channel.lvclass"=w5525, "Acquisition in"=w5522) -> ("error out"=w5524:errorcluster, "Acquisition out"=w5523:refnum<class "Acquisition.lvclass">)  [unwired: 7 in]
            }
          }
          n1971 = call-dynamic "Write AcquisitionC.vi"("error in (no error)"=w5469, "Acquisition.lvclass"=w5467, "S4ACS_GUI in"=w5468) -> ("error out"=w5445:errorcluster, "S4ACS_GUI out"=w5461:refnum<class "S4GUI.lvclass">)  [unwired: 7 in]
          n1972 = call-dynamic "Read AcquisitionD.vi"("error in (no error)"=w5445, "S4ACS_GUI in"=w5461) -> ("error out"=w5441:errorcluster, "Acquisition.lvclass"=w5444:refnum<class "Acquisition.lvclass">, "S4ACS_GUI out"=w5463:refnum<class "S4GUI.lvclass">)  [unwired: 7 in]
          n1973 = call-dynamic "Read enabled.vi"("error in (no error)"=w5441, "Server in"=w5444) -> ("error out"=w5442:errorcluster, "enabled"=w5440:bool, "Server out"=w5443:refnum<class "Acquisition.lvclass">)  [unwired: 7 in]
          n1974 = case shown="True" w5440 {
            tunnel: [w5485 w5504] -> w5464
            tunnel: [w5484 w5503] -> w5462
            tunnel: [TRUE w5492] -> w5435
            tunnel: w5443 -> [w5485 w5495]
            tunnel: w5442 -> [w5484 w5494]
            tunnel: [u32 0 ("CyclesDone") w5486] -> w5428
            frame False {
            }
            frame True {
              n1975 = call-dynamic "Read Channel.vi"("error in (no error)"=w5494, "Acquisition in"=w5495) -> ("error out"=w5488:errorcluster, "Channel.lvclass"=w5490:refnum<class "Channel.lvclass">, "Acquisition out"=w5505:refnum<class "Acquisition.lvclass">)  [unwired: 7 in]
              n1976 = call-dynamic "Read CyclesDone.vi"("error in (no error)"=w5488, "Channel in"=w5490) -> ("error out"=w5487:errorcluster, "CyclesDone"=w5486:u32, "Channel out"=w5489:refnum<class "Channel.lvclass">)  [unwired: 7 in]
              n1977 = call-dynamic "Read State Machine.vi"("error in (no error)"=w5487, "Device in"=w5489) -> ("error out"=w5497:errorcluster, "State Machine.lvclass"=w5499:refnum<class "State Machine.lvclass">, "Device out"=w5501:refnum<class "Channel.lvclass">)  [unwired: 7 in]
              n1978 = call-dynamic "Read State.vi"("error in (no error)"=w5497, "State Machine in"=w5499) -> ("error out"=w5496:errorcluster, "State"=w5491:i32, "State Machine out"=w5498:refnum<class "State Machine.lvclass">)  [unwired: 7 in]
              n1979 = Greater?(x=w5491, y=53) -> (0:w5492:bool)
              n1980 = call-dynamic "Write State Machine.vi"("error in (no error)"=w5496, "State Machine.lvclass"=w5498, "Device in"=w5501) -> ("error out"=w5500:errorcluster, "Device out"=w5502:refnum<class "Channel.lvclass">)  [unwired: 7 in]
              n1981 = call-dynamic "Write Channel.vi"("error in (no error)"=w5500, "Channel.lvclass"=w5502, "Acquisition in"=w5505) -> ("error out"=w5503:errorcluster, "Acquisition out"=w5504:refnum<class "Acquisition.lvclass">)  [unwired: 7 in]
            }
          }
          n1982 = call-dynamic "Write AcquisitionD.vi"("error in (no error)"=w5462, "Acquisition.lvclass"=w5464, "S4ACS_GUI in"=w5463) -> ("error out"=w5433:errorcluster, "S4ACS_GUI out"=w5434:refnum<class "S4GUI.lvclass">)  [unwired: 7 in]
          n1983 = Compound Arithmetic op=AND(w5438, w5437, w5436, w5435) -> ()  [unwired: 1 out]
          n1984 = Compound Arithmetic op=ADD(w5430, w5431, w5429, w5428) -> (w5427:u32)
          n1985 = Equal To 0?(x=w5427) -> (x = 0?=w5426:bool)
          n1986 = Increment(x=w5439) -> (x+1=w5432:u32)
          n1987 = Select(t=w5432, s=w5426, f=w5439) -> (s? t:f=w5475:u32)
          n1988 = Bundle By Name(cluster=w5434, "Obs_state"=w5475) -> (w5476:refnum<class "S4GUI.lvclass">)
        }
        frame 367 {
          # "T=canais receberam STOP"
          # "OV 2024.01.26 DEBUG - ignora os ciclos!!\nT= Todos os canais ativos no mesmo ciclo;\nF= Canais com ciclo diferente"
          # "T= Todos os canais ativos na mesma sequencia;\nF= Canais com sequencia diferente"
          # "Todos os CYCLES_DONE \nmudaram e são iguais?\nSe sim, avança a lâmina."
          n1989 = Unbundle By Name(w5613) -> ("cyclesDone"=w5607:u32)
          n1990 = call-dynamic "Read AcquisitionA.vi"("error in (no error)"=w5648, "S4ACS_GUI in"=w5613) -> ("error out"=w5628:errorcluster, "Acquisition.lvclass"=w5629:refnum<class "Acquisition.lvclass">, "S4ACS_GUI out"=w5650:refnum<class "S4GUI.lvclass">)  [unwired: 7 in]
          n1991 = call-dynamic "Read enabled.vi"("error in (no error)"=w5628, "Server in"=w5629) -> ("error out"=w5627:errorcluster, "enabled"=w5595:bool, "Server out"=w5626:refnum<class "Acquisition.lvclass">)  [unwired: 7 in]
          n1992 = case shown="True" w5595 {
            tunnel: w5627 -> [w5865 w5884]
            tunnel: [w5866 w5882] -> w5651
            tunnel: [w5865 w5881] -> w5649
            tunnel: [u32 0 ("SequesDone") w5880] -> w5601
            tunnel: w5626 -> [w5866 w5879]
            tunnel: w5607 -> [_ w5878]
            tunnel: [TRUE w5877] -> w5612
            tunnel: [u32 0 ("CubesDone") w5876] -> w5588
            tunnel: [FALSE ("stopping") w5867] -> w5584
            frame False {
            }
            frame True {
              # "CYCLES_DONE = 0->1"
              n1993 = call-dynamic "Read Channel.vi"("error in (no error)"=w5884, "Acquisition in"=w5879) -> ("error out"=w5873:errorcluster, "Channel.lvclass"=w5875:refnum<class "Channel.lvclass">, "Acquisition out"=w5883:refnum<class "Acquisition.lvclass">)  [unwired: 7 in]
              n1994 = call-dynamic "Read CyclesDone.vi"("error in (no error)"=w5873, "Channel in"=w5875) -> ("error out"=w5872:errorcluster, "CyclesDone"=w5876:u32, "Channel out"=w5874:refnum<class "Channel.lvclass">)  [unwired: 7 in]
              n1995 = call-dynamic "Read CyclesDone.vi"("error in (no error)"=w5872, "Channel in"=w5874) -> ("error out"=w5870:errorcluster, "CyclesDone"=w5880:u32, "Channel out"=w5871:refnum<class "Channel.lvclass">)  [unwired: 7 in]
              n1996 = Not Equal?(x=w5880, y=w5878) -> (x != y?=w5877:bool)
              n1997 = call-dynamic "Read stopping.vi"("error in (no error)"=w5870, "Channel in"=w5871) -> ("error out"=w5869:errorcluster, "stopping"=w5867:bool, "Channel out"=w5868:refnum<class "Channel.lvclass">)  [unwired: 7 in]
              n1998 = call-dynamic "Write Channel.vi"("error in (no error)"=w5869, "Channel.lvclass"=w5868, "Acquisition in"=w5883) -> ("error out"=w5881:errorcluster, "Acquisition out"=w5882:refnum<class "Acquisition.lvclass">)  [unwired: 7 in]
            }
          }
          n1999 = call-dynamic "Write AcquisitionA.vi"("error in (no error)"=w5649, "Acquisition.lvclass"=w5651, "S4ACS_GUI in"=w5650) -> ("error out"=w5645:errorcluster, "S4ACS_GUI out"=w5644:refnum<class "S4GUI.lvclass">)  [unwired: 7 in]
          n2000 = call "Read AcquisitionB.vi"("error in (no error)"=w5645, "S4ACS_GUI in"=w5644) -> ("error out"=w5622:errorcluster, "Acquisition.lvclass"=w5625:refnum<class "Acquisition.lvclass">, "S4ACS_GUI out"=w5646:refnum<class "S4GUI.lvclass">)  [unwired: 7 in]
          n2001 = call-dynamic "Read enabled.vi"("error in (no error)"=w5622, "Server in"=w5625) -> ("error out"=w5623:errorcluster, "enabled"=w5594:bool, "Server out"=w5624:refnum<class "Acquisition.lvclass">)  [unwired: 7 in]
          n2002 = case shown="True" w5594 {
            tunnel: w5623 -> [w5841 w5860]
            tunnel: w5624 -> [w5842 w5859]
            tunnel: [u32 0 ("SequesDone") w5854] -> w5598
            tunnel: [w5841 w5858] -> w5643
            tunnel: [w5842 w5857] -> w5642
            tunnel: w5607 -> [_ w5853]
            tunnel: [TRUE w5852] -> w5608
            tunnel: [u32 0 ("CubesDone") w5847] -> w5587
            tunnel: [FALSE ("stopping") w5843] -> w5583
            frame False {
            }
            frame True {
              n2003 = call-dynamic "Read Channel.vi"("error in (no error)"=w5860, "Acquisition in"=w5859) -> ("error out"=w5849:errorcluster, "Channel.lvclass"=w5851:refnum<class "Channel.lvclass">, "Acquisition out"=w5855:refnum<class "Acquisition.lvclass">)  [unwired: 7 in]
              n2004 = call-dynamic "Read CyclesDone.vi"("error in (no error)"=w5849, "Channel in"=w5851) -> ("error out"=w5848:errorcluster, "CyclesDone"=w5847:u32, "Channel out"=w5850:refnum<class "Channel.lvclass">)  [unwired: 7 in]
              n2005 = call-dynamic "Read CyclesDone.vi"("error in (no error)"=w5848, "Channel in"=w5850) -> ("error out"=w5845:errorcluster, "CyclesDone"=w5854:u32, "Channel out"=w5856:refnum<class "Channel.lvclass">)  [unwired: 7 in]
              n2006 = Not Equal?(x=w5854, y=w5853) -> (x != y?=w5852:bool)
              n2007 = call-dynamic "Read stopping.vi"("error in (no error)"=w5845, "Channel in"=w5856) -> ("error out"=w5844:errorcluster, "stopping"=w5843:bool, "Channel out"=w5846:refnum<class "Channel.lvclass">)  [unwired: 7 in]
              n2008 = call-dynamic "Write Channel.vi"("error in (no error)"=w5844, "Channel.lvclass"=w5846, "Acquisition in"=w5855) -> ("error out"=w5858:errorcluster, "Acquisition out"=w5857:refnum<class "Acquisition.lvclass">)  [unwired: 7 in]
            }
          }
          n2009 = Max & Min(x=w5588, y=w5587) -> (max(x,y)=w5604:u32)  [unwired: 1 out]
          n2010 = Max & Min(x=w5601, y=w5598) -> (max(x,y)=w5611:u32)  [unwired: 1 out]
          n2011 = call "Write AcquisitionB.vi"("error in (no error)"=w5643, "Acquisition.lvclass"=w5642, "S4ACS_GUI in"=w5646) -> ("error out"=w5635:errorcluster, "S4ACS_GUI out"=w5634:refnum<class "S4GUI.lvclass">)  [unwired: 7 in]
          n2012 = call-dynamic "Read AcquisitionC.vi"("error in (no error)"=w5635, "S4ACS_GUI in"=w5634) -> ("error out"=w5619:errorcluster, "Acquisition.lvclass"=w5621:refnum<class "Acquisition.lvclass">, "S4ACS_GUI out"=w5637:refnum<class "S4GUI.lvclass">)  [unwired: 7 in]
          n2013 = call-dynamic "Read enabled.vi"("error in (no error)"=w5619, "Server in"=w5621) -> ("error out"=w5618:errorcluster, "enabled"=w5593:bool, "Server out"=w5620:refnum<class "Acquisition.lvclass">)  [unwired: 7 in]
          n2014 = case shown="True" w5593 {
            tunnel: [w5817 w5836] -> w5638
            tunnel: [w5818 w5835] -> w5636
            tunnel: w5618 -> [w5817 w5832]
            tunnel: w5620 -> [w5818 w5833]
            tunnel: [u32 0 ("SequesDone") w5831] -> w5597
            tunnel: w5607 -> [_ w5830]
            tunnel: [TRUE w5829] -> w5606
            tunnel: [u32 0 ("CubesDone") w5823] -> w5586
            tunnel: [FALSE ("stopping") w5819] -> w5582
            frame False {
            }
            frame True {
              n2015 = call-dynamic "Read Channel.vi"("error in (no error)"=w5832, "Acquisition in"=w5833) -> ("error out"=w5825:errorcluster, "Channel.lvclass"=w5827:refnum<class "Channel.lvclass">, "Acquisition out"=w5834:refnum<class "Acquisition.lvclass">)  [unwired: 7 in]
              n2016 = call-dynamic "Read CyclesDone.vi"("error in (no error)"=w5825, "Channel in"=w5827) -> ("error out"=w5824:errorcluster, "CyclesDone"=w5823:u32, "Channel out"=w5826:refnum<class "Channel.lvclass">)  [unwired: 7 in]
              n2017 = call-dynamic "Read CyclesDone.vi"("error in (no error)"=w5824, "Channel in"=w5826) -> ("error out"=w5821:errorcluster, "CyclesDone"=w5831:u32, "Channel out"=w5828:refnum<class "Channel.lvclass">)  [unwired: 7 in]
              n2018 = Not Equal?(x=w5831, y=w5830) -> (x != y?=w5829:bool)
              n2019 = call-dynamic "Read stopping.vi"("error in (no error)"=w5821, "Channel in"=w5828) -> ("error out"=w5820:errorcluster, "stopping"=w5819:bool, "Channel out"=w5822:refnum<class "Channel.lvclass">)  [unwired: 7 in]
              n2020 = call-dynamic "Write Channel.vi"("error in (no error)"=w5820, "Channel.lvclass"=w5822, "Acquisition in"=w5834) -> ("error out"=w5836:errorcluster, "Acquisition out"=w5835:refnum<class "Acquisition.lvclass">)  [unwired: 7 in]
            }
          }
          n2021 = call-dynamic "Write AcquisitionC.vi"("error in (no error)"=w5638, "Acquisition.lvclass"=w5636, "S4ACS_GUI in"=w5637) -> ("error out"=w5632:errorcluster, "S4ACS_GUI out"=w5633:refnum<class "S4GUI.lvclass">)  [unwired: 7 in]
          n2022 = call-dynamic "Read AcquisitionD.vi"("error in (no error)"=w5632, "S4ACS_GUI in"=w5633) -> ("error out"=w5615:errorcluster, "Acquisition.lvclass"=w5617:refnum<class "Acquisition.lvclass">, "S4ACS_GUI out"=w5639:refnum<class "S4GUI.lvclass">)  [unwired: 7 in]
          n2023 = call-dynamic "Read enabled.vi"("error in (no error)"=w5615, "Server in"=w5617) -> ("error out"=w5614:errorcluster, "enabled"=w5592:bool, "Server out"=w5616:refnum<class "Acquisition.lvclass">)  [unwired: 7 in]
          n2024 = Build Array(w5595, w5594, w5593, w5592) -> (w5591:bool[])
          n2025 = case shown="True" w5592 {
            tunnel: [w5794 w5812] -> w5641
            tunnel: [w5793 w5811] -> w5640
            tunnel: w5616 -> [w5794 w5810]
            tunnel: w5614 -> [w5793 w5809]
            tunnel: [u32 0 ("SequesDone") w5807] -> w5600
            tunnel: w5607 -> [_ w5806]
            tunnel: [TRUE w5805] -> w5605
            tunnel: [u32 0 ("CubesDone") w5799] -> w5585
            tunnel: [FALSE ("stopping") w5795] -> w5581
            frame False {
            }
            frame True {
              n2026 = call-dynamic "Read Channel.vi"("error in (no error)"=w5809, "Acquisition in"=w5810) -> ("error out"=w5801:errorcluster, "Channel.lvclass"=w5803:refnum<class "Channel.lvclass">, "Acquisition out"=w5808:refnum<class "Acquisition.lvclass">)  [unwired: 7 in]
              n2027 = call-dynamic "Read CyclesDone.vi"("error in (no error)"=w5801, "Channel in"=w5803) -> ("error out"=w5800:errorcluster, "CyclesDone"=w5799:u32, "Channel out"=w5802:refnum<class "Channel.lvclass">)  [unwired: 7 in]
              n2028 = call-dynamic "Read CyclesDone.vi"("error in (no error)"=w5800, "Channel in"=w5802) -> ("error out"=w5797:errorcluster, "CyclesDone"=w5807:u32, "Channel out"=w5804:refnum<class "Channel.lvclass">)  [unwired: 7 in]
              n2029 = Not Equal?(x=w5807, y=w5806) -> (x != y?=w5805:bool)
              n2030 = call-dynamic "Read stopping.vi"("error in (no error)"=w5797, "Channel in"=w5804) -> ("error out"=w5796:errorcluster, "stopping"=w5795:bool, "Channel out"=w5798:refnum<class "Channel.lvclass">)  [unwired: 7 in]
              n2031 = call-dynamic "Write Channel.vi"("error in (no error)"=w5796, "Channel.lvclass"=w5798, "Acquisition in"=w5808) -> ("error out"=w5811:errorcluster, "Acquisition out"=w5812:refnum<class "Acquisition.lvclass">)  [unwired: 7 in]
            }
          }
          n2032 = Boolean Array To Number(Boolean array=w5591) -> (number=w5589:u32)
          n2033 = Max & Min(x=w5586, y=w5585) -> (max(x,y)=w5603:u32)  [unwired: 1 out]
          n2034 = Max & Min(x=w5597, y=w5600) -> (max(x,y)=w5610:u32)  [unwired: 1 out]
          n2035 = Compound Arithmetic op=AND(w5612, w5608, w5606, w5605) -> (w5590:bool)
          n2036 = Max & Min(x=w5611, y=w5610) -> (max(x,y)=w5609:u32)  [unwired: 1 out]
          n2037 = Max & Min(x=w5604, y=w5603) -> (max(x,y)=w5602:u32)  [unwired: 1 out]
          n2038 = case shown="12" w5589 {
            tunnel: w5588 -> [w5659 _ w5671 _ w5680 _ w5686 w5692 _ w5698 w5701 _]
            tunnel: w5585 -> [w5658 w5662 w5667 w5674 w5675 w5683 w5685 _ _ _ _ _]
            tunnel: w5587 -> [w5657 w5660 _ _ w5679 w5681 _ w5691 w5695 _ w5700 _]
            tunnel: w5586 -> [w5656 w5661 w5666 w5672 _ _ _ w5690 w5694 w5697 _ _]
            tunnel: [w5652 w5663 w5668 w5673 w5676 w5682 w5684 w5687 w5693 w5696 w5699 TRUE] -> _
            frame 15 {
              # "A,B,C,D ativos"
              n2039 = Equal?(x=w5659, y=w5657) -> (x = y?=w5655:bool)
              n2040 = Equal?(x=w5656, y=w5658) -> (x = y?=w5653:bool)
              n2041 = Equal?(x=w5657, y=w5656) -> (x = y?=w5654:bool)
              n2042 = Compound Arithmetic op=AND(w5655, w5654, w5653) -> (w5652:bool)
            }
            frame 14 {
              # "B,C e,D ativos"
              n2043 = Equal?(x=w5660, y=w5661) -> (x = y?=w5665:bool)
              n2044 = Equal?(x=w5661, y=w5662) -> (x = y?=w5664:bool)
              n2045 = Compound Arithmetic op=AND(w5665, w5664) -> (w5663:bool)
            }
            frame 13 {
              # "A,C e,D ativos"
              n2046 = Equal?(x=w5671, y=w5666) -> (x = y?=w5670:bool)
              n2047 = Equal?(x=w5666, y=w5667) -> (x = y?=w5669:bool)
              n2048 = Compound Arithmetic op=AND(w5670, w5669) -> (w5668:bool)
            }
            frame 12 {
              # "Só C e D ativos"
              n2049 = Equal?(x=w5672, y=w5674) -> (x = y?=w5673:bool)
            }
            frame 11 {
              # "A,B e,D ativos"
              n2050 = Equal?(x=w5680, y=w5679) -> (x = y?=w5678:bool)
              n2051 = Equal?(x=w5679, y=w5675) -> (x = y?=w5677:bool)
              n2052 = Compound Arithmetic op=AND(w5678, w5677) -> (w5676:bool)
            }
            frame 10 {
              # "Só B e D ativos"
              n2053 = Equal?(x=w5681, y=w5683) -> (x = y?=w5682:bool)
            }
            frame 9 {
              # "Só A e D ativos"
              n2054 = Equal?(x=w5686, y=w5685) -> (x = y?=w5684:bool)
            }
            frame 7 {
              # "A,B,C ativos"
              n2055 = Equal?(x=w5692, y=w5691) -> (x = y?=w5689:bool)
              n2056 = Equal?(x=w5691, y=w5690) -> (x = y?=w5688:bool)
              n2057 = Compound Arithmetic op=AND(w5689, w5688) -> (w5687:bool)
            }
            frame 6 {
              # "Só B e C ativos"
              n2058 = Equal?(x=w5695, y=w5694) -> (x = y?=w5693:bool)
            }
            frame 5 {
              # "Só A e C ativos"
              n2059 = Equal?(x=w5698, y=w5697) -> (x = y?=w5696:bool)
            }
            frame 3 {
              # "só A e B ativos"
              n2060 = Equal?(x=w5701, y=w5700) -> (x = y?=w5699:bool)
            }
            frame 0..2, 4, 8, Default {
              # "nenhum ou só 1  \ncanal ativo."
            }
          }
          n2061 = Compound Arithmetic op=OR(w5584, w5583, w5582, w5581) -> (w5580:bool)
          n2062 = case shown="0..2, 4, 8, Default" w5589 {
            tunnel: w5601 -> [w5710 _ w5722 _ w5731 _ w5737 w5743 _ w5749 w5752 _]
            tunnel: w5600 -> [w5709 w5713 w5718 w5725 w5726 w5734 w5736 _ _ _ _ _]
            tunnel: w5598 -> [w5708 w5711 _ _ w5730 w5732 _ w5742 w5746 _ w5751 _]
            tunnel: w5597 -> [w5707 w5712 w5717 w5723 _ _ _ w5741 w5745 w5748 _ _]
            tunnel: [w5703 w5714 w5719 w5724 w5727 w5733 w5735 w5738 w5744 w5747 w5750 TRUE] -> w5596
            frame 15 {
              # "A,B,C,D ativos"
              n2063 = Equal?(x=w5710, y=w5708) -> (x = y?=w5706:bool)
              n2064 = Equal?(x=w5707, y=w5709) -> (x = y?=w5704:bool)
              n2065 = Equal?(x=w5708, y=w5707) -> (x = y?=w5705:bool)
              n2066 = Compound Arithmetic op=AND(w5706, w5705, w5704) -> (w5703:bool)
            }
            frame 14 {
              # "B,C e,D ativos"
              n2067 = Equal?(x=w5711, y=w5712) -> (x = y?=w5716:bool)
              n2068 = Equal?(x=w5712, y=w5713) -> (x = y?=w5715:bool)
              n2069 = Compound Arithmetic op=AND(w5716, w5715) -> (w5714:bool)
            }
            frame 13 {
              # "A,C e,D ativos"
              n2070 = Equal?(x=w5722, y=w5717) -> (x = y?=w5721:bool)
              n2071 = Equal?(x=w5717, y=w5718) -> (x = y?=w5720:bool)
              n2072 = Compound Arithmetic op=AND(w5721, w5720) -> (w5719:bool)
            }
            frame 12 {
              # "Só C e D ativos"
              n2073 = Equal?(x=w5723, y=w5725) -> (x = y?=w5724:bool)
            }
            frame 11 {
              # "A,B e,D ativos"
              n2074 = Equal?(x=w5731, y=w5730) -> (x = y?=w5729:bool)
              n2075 = Equal?(x=w5730, y=w5726) -> (x = y?=w5728:bool)
              n2076 = Compound Arithmetic op=AND(w5729, w5728) -> (w5727:bool)
            }
            frame 10 {
              # "Só B e D ativos"
              n2077 = Equal?(x=w5732, y=w5734) -> (x = y?=w5733:bool)
            }
            frame 9 {
              # "Só A e D ativos"
              n2078 = Equal?(x=w5737, y=w5736) -> (x = y?=w5735:bool)
            }
            frame 7 {
              # "A,B,C ativos"
              n2079 = Equal?(x=w5743, y=w5742) -> (x = y?=w5740:bool)
              n2080 = Equal?(x=w5742, y=w5741) -> (x = y?=w5739:bool)
              n2081 = Compound Arithmetic op=AND(w5740, w5739) -> (w5738:bool)
            }
            frame 6 {
              # "Só B e C ativos"
              n2082 = Equal?(x=w5746, y=w5745) -> (x = y?=w5744:bool)
            }
            frame 5 {
              # "Só A e C ativos"
              n2083 = Equal?(x=w5749, y=w5748) -> (x = y?=w5747:bool)
            }
            frame 3 {
              # "só A e B ativos"
              n2084 = Equal?(x=w5752, y=w5751) -> (x = y?=w5750:bool)
            }
            frame 0..2, 4, 8, Default {
              # "nenhum ou só 1  \ncanal ativo."
            }
          }
          n2085 = call-dynamic "Write AcquisitionD.vi"("error in (no error)"=w5640, "Acquisition.lvclass"=w5641, "S4ACS_GUI in"=w5639) -> ("error out"=w5630:errorcluster, "S4ACS_GUI out"=w5631:refnum<class "S4GUI.lvclass">)  [unwired: 7 in]
          n2086 = And(x=w5590, y=w5596) -> (x .and. y?=w5599:bool)
          n2087 = case shown="True" w5599 {
            tunnel: w5631 -> [w5755 w5767]
            tunnel: [w5754 w5766] -> w5647
            tunnel: w5609 -> [_ w5765]
            tunnel: w5602 -> [_ _]
            tunnel: w5590 -> [w5756 _]
            tunnel: TRUE -> [_ w5764]
            tunnel: w5580 -> [_ w5763]
            tunnel: w5578 -> [_ w5762]
            frame False {
              n2088 = case shown="True" w5756 {
                tunnel: w5755 -> [w5757 w5761]
                tunnel: [w5757 w5760] -> w5754
                frame False {
                }
                frame True {
                  n2089 = Bundle By Name(cluster=w5761, "Obs_state"=u32 1, "Error Msg"="ERROR: Sequence_done not equal in all active channels.") -> (w5760:refnum<class "S4GUI.lvclass">)
                }
              }
            }
            frame True {
              n2090 = case shown="True" w5764 {
                tunnel: w5767 -> [w5769 w5779]
                tunnel: [w5768 w5778] -> w5766
                tunnel: w5765 -> [_ w5777]
                tunnel: w5763 -> [_ w5773]
                tunnel: w5762 -> [_ w5772]
                frame False {
                  n2091 = Bundle By Name(cluster=w5769, "Obs_state"=u32 1, "Error Msg"="ERROR: Cycles_done not equal in all active channels.") -> (w5768:refnum<class "S4GUI.lvclass">)
                }
                frame True {
                  # "STOP?"
                  n2092 = local read "time308"() -> (w5775:u32)
                  n2093 = Tick Count (ms)() -> (millisecond timer value=w5776:u32)
                  n2094 = Subtract(x=w5776, y=w5775) -> (x-y=→"delay Acq 2":u32)
                  n2095 = case shown="False" w5773 {
                    tunnel: w5779 -> [w5783 w5788]
                    tunnel: [w5782 w5787] -> w5778
                    tunnel: w5777 -> [w5780 w5784]
                    tunnel: w5772 -> [_ w5786]
                    frame True {
                      n2096 = Bundle By Name(cluster=w5783, "Obs_state"=u32 0, "sequesDone"=w5780, "cyclesDone"=w5780) -> (w5782:refnum<class "S4GUI.lvclass">)
                    }
                    frame False {
                      n2097 = Increment(x=w5786) -> (x+1=w5785:u32)
